vi "fgv_Gslam_history.vi"(7 "cmd":enum16{"ini", "add hxTrue-DR", "add z", "read"}(ring), 9 "z":dbl[][](array[numeric]), 10 "x_dr":cluster{"x":dbl, "y":dbl, "yaw":dbl}, 11 "x_true":cluster{"x":dbl, "y":dbl, "yaw":dbl}) -> (1 "hz":dbl[][][](array[numeric]), 2 "hxDR":cluster{"x":dbl, "y":dbl, "yaw":dbl}[](array[cluster]), 3 "hxTrue":cluster{"x":dbl, "y":dbl, "yaw":dbl}[](array[cluster]))   [LabVIEW 2019]
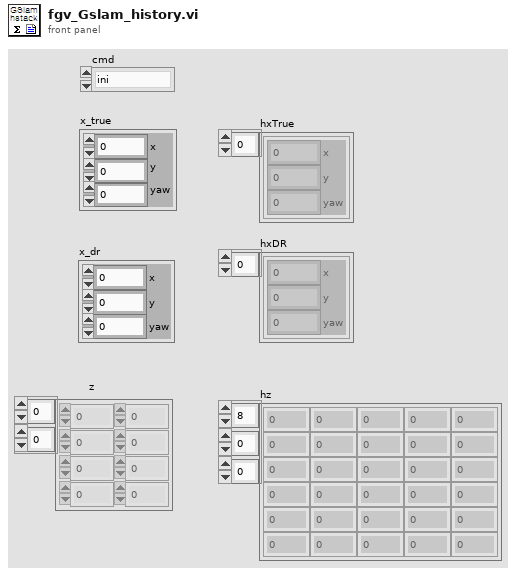
[diagram p1: front panel]
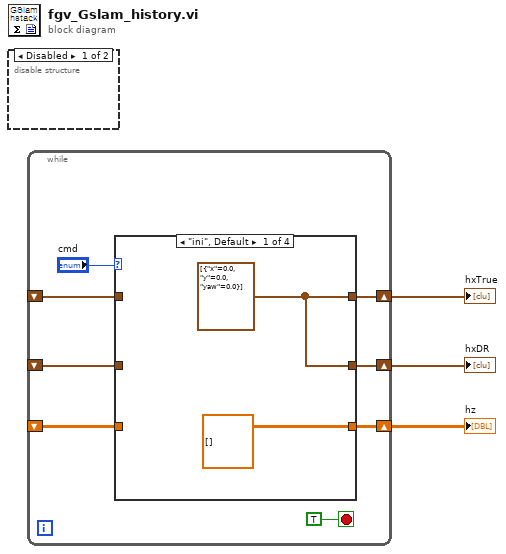
[diagram p0: block diagram]
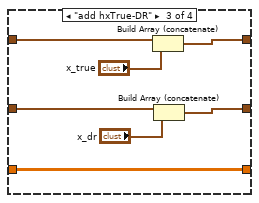
[diagram p4: hidden frame]
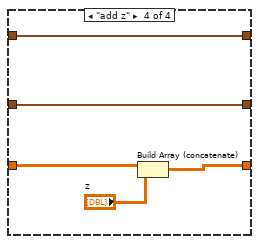
[diagram p5: hidden frame]
diagram:
  n1 = disable-structure shown="Disabled" {
    frame Disabled {
    }
    frame Enabled {
    }
  }
  n2 = while {
    shift-right: [w10] -> w2
    shift-left: _ -> [w7]
    shift-right: [w9] -> w1
    shift-left: _ -> [w6]
    shift-right: [w8] -> w3
    shift-left: _ -> [w5]
    stop <- TRUE stop-if-true
    n3 = case shown="\"ini\", Default" "cmd" {
      tunnel: [w13 w16 w21 w28] -> w10
      tunnel: [w13 w15 w19 w27] -> w9
      tunnel: [dbl[][][] [] w14 w17 w25] -> w8
      tunnel: w7 -> [_ w16 w23 w28]
      tunnel: w6 -> [_ w15 w20 w27]
      tunnel: w5 -> [_ w14 w17 w24]
      frame "ini", Default {
        w13 = cluster{"x":dbl, "y":dbl, "yaw":dbl}[] [{"x"=0.0, "y"=0.0, "yaw"=0.0}]
      }
      frame "read" {
      }
      frame "add hxTrue-DR" {
        n4 = Build Array (concatenate)(w23, "x_true") -> (w21:cluster{"x":dbl, "y":dbl, "yaw":dbl}[])
        n5 = Build Array (concatenate)(w20, "x_dr") -> (w19:cluster{"x":dbl, "y":dbl, "yaw":dbl}[])
      }
      frame "add z" {
        n6 = Build Array (concatenate)(w24, "z") -> (w25:dbl[][][])
      }
    }
  }
  "hz" <- w3
  "hxTrue" <- w2
  "hxDR" <- w1
